vi "BRig_dataExp_Loop_T_Cue.vi"() -> (2 "output_Loop_T_Cue":i32)   [LabVIEW 2014]
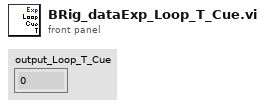
[diagram p1: front panel]
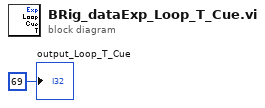
[diagram p0: block diagram]
diagram:
  "output_Loop_T_Cue" <- 69 ("output_iBlock")
